vi "Extract embedded cluster control refs.vi"(8 "error in (no error)":errorcluster, 11 "Controls IN":refnum<vi>[](array[refnum])) -> (0 "error out":errorcluster, 3 "Controls OUT":refnum<vi>[](array[refnum]))   [LabVIEW 2017]
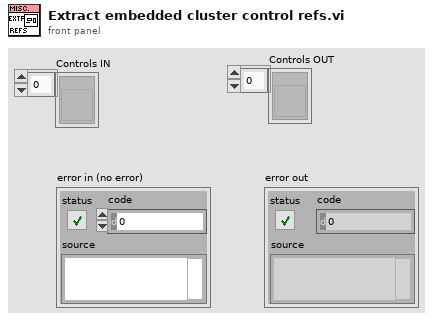
[diagram p1: front panel]
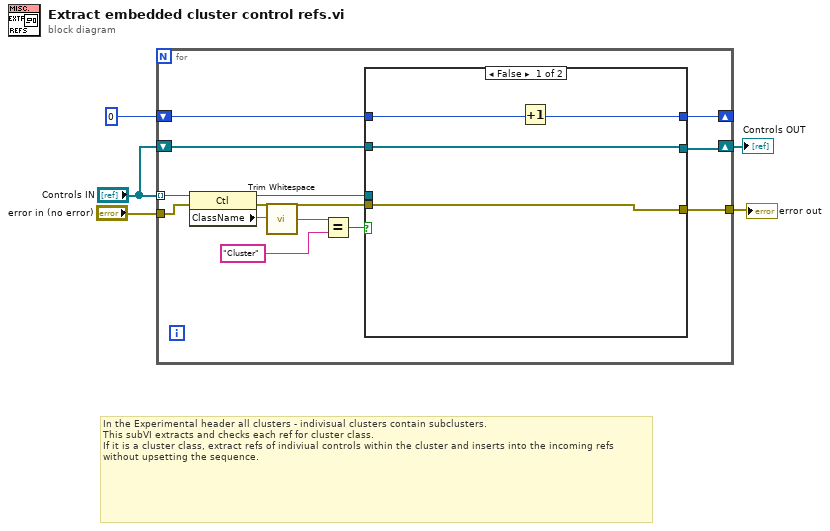
[diagram p0: block diagram]
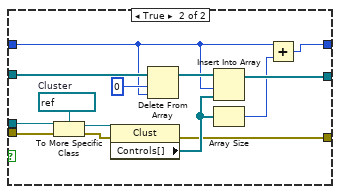
[diagram p2: hidden frame]
diagram:
  # "In the Experimental header all clusters - indivisual clusters contain subclusters.\nThis subVI extracts and checks each ref for cluster class.\nIf it is a cluster class, extract refs of indiviual controls within the cluster and inserts into the incoming refs\nwithout upsetting the sequence."
  n1 = for {
    tunnel: "Controls IN" -> [w18] mode=indexing
    shift-right: [w11] -> w3
    shift-left: "Controls IN" -> [w12]
    shift-right: [w10] -> _
    shift-left: 0 -> [w9]
    tunnel: "error in (no error)" -> [w8]
    tunnel: [w6] -> w1
    n2 = property class="Ctl"(reference=w18, error in=w8) -> (reference out=w13:refnum<vi>, error out=w7:errorcluster, "ClassName"=w17:string)
    n3 = call <vilib>:"Trim Whitespace.vi"("string"=w17) -> ("trimmed string"=w16:string)  [unwired: 1 in]
    n4 = Equal?(x=w16, y="Cluster") -> (x = y?=w14:bool)
    n5 = case shown="False" w14 {
      tunnel: w13 -> [_ w36]
      tunnel: w12 -> [w22 w33]
      tunnel: [w22 w30] -> w11
      tunnel: [w21 w26] -> w10
      tunnel: w9 -> [w20 w29]
      tunnel: w7 -> [w19 w25]
      tunnel: [w19 w23] -> w6
      frame False {
        n6 = Increment(x=w20) -> (x+1=w21:i32)
      }
      frame True {
        w35 = refnum<vi> refnum  # Cluster
        n7 = To More Specific Class(target class=w35, reference=w36, error in=w25) -> (specific class reference=w34:refnum<vi>, error out=w24:errorcluster)
        n8 = property class="Clust"(reference=w34, error in=w24) -> (error out=w23:errorcluster, "Controls[]"=w28:refnum<vi>[])  [unwired: 1 out]
        n9 = Delete From Array(array=w33, length=0, index=w29) -> (array with subset deleted=w31:refnum<vi>[])  [unwired: 1 out]
        n10 = Insert Into Array(array=w31, index=w29, new element=w28) -> (w30:refnum<vi>[])
        n11 = Array Size(array=w28) -> (size(s)=w27:i32)
        n12 = Add(x=w29, y=w27) -> (x+y=w26:i32)
      }
    }
  }
  "Controls OUT" <- w3
  "error out" <- w1
